vi "Test for Stage class.vi"(8 "error in":errorcluster, 9 "INI File Path":path=path "C:/AME Test Engineering/LabVIEW/PPLs/Axis/Thorlabs KBD/config.ini", 10 "PPLs Folder Path":path=path "C:/AME Test Engineering/LabVIEW/PPLs", 11 "Device":string="Axis") -> (0 "error out":errorcluster)   [LabVIEW 2018]
uses:
  Parent/Axis.lvlibp/Axis.lvclass
panel:
  out "error out 2":errorcluster
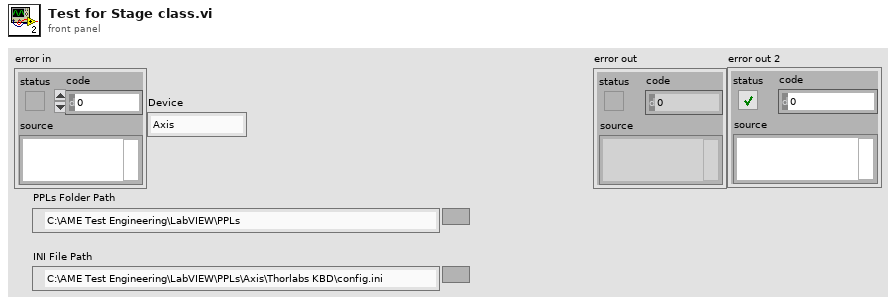
[diagram p1: front panel]
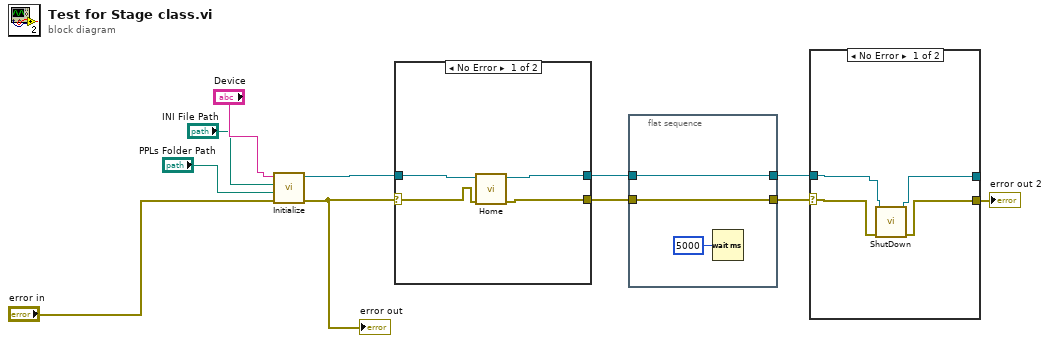
[diagram p0: block diagram]
diagram:
  n1 = call "Initialize.vi"("error in"="error in", "PPLs Folder Path"="PPLs Folder Path", "INI File Path"="INI File Path", "Device"="Device") -> ("error out"=w5:errorcluster, "Axis out"=w4:refnum<class "Axis.lvclass">)  [unwired: 6 in]
  "error out" <- w5
  n2 = case shown="No Error" w5 {
    selector: w5 -> [w13 w16]
    tunnel: w4 -> [w15 w17]
    tunnel: [w14 w17] -> w11
    tunnel: [w12 w16] -> w10
    frame No Error {
      n3 = call "Home.vi"("error in"=w13, "Axis in"=w15) -> ("error out"=w12:errorcluster, "Axis out"=w14:refnum<class "Axis.lvclass">)  [unwired: 7 in, 1 out]
    }
    frame Error {
    }
  }
  n4 = flat-sequence {
    tunnel: w11 -> [w19]
    tunnel: w10 -> [w18]
    tunnel: [w19] -> w8
    tunnel: [w18] -> w9
    frame #0 {
      n5 = Wait (ms)(milliseconds to wait=u32 5000) -> ()  [unwired: 1 out]
    }
  }
  n6 = case shown="No Error" w9 {
    selector: w9 -> [w23 w25]
    tunnel: w8 -> [w24 w26]
    tunnel: [w21 w26] -> _
    tunnel: [w22 w25] -> w7
    frame No Error {
      n7 = call "ShutDown.vi"("error in"=w23, "Axis in"=w24) -> ("error out"=w22:errorcluster, "Axis out"=w21:refnum<class "Axis.lvclass">)  [unwired: 8 in]
    }
    frame Error {
    }
  }
  "error out 2" <- w7
